vi "reward_behavior_0_6s_post_stim_timeout.vi"() -> ()   [LabVIEW 2019]
doc: "The myRIO Project template acquires acceleration data from the onboard accelerometer and displays the changes of acceleration values in a waveform chart."
uses:
  <vilib>/Analysis/Matrix/Datatypes/RealMatrix.ctl
  <vilib>/myRIO/Common/Instrument Driver Framework/myRIO v1.0/Encoder/typedefs/Encoder Signal Mode.ctl
  <vilib>/myRIO/Instrument Drivers/Onboard IO/Encoder/typedefs/Encoder Reference.ctl
  <vilib>/myRIO/Common/Instrument Driver Framework/Utilities/typedefs/myRIO Generic Hardware Reference.ctl
  <vilib>/myRIO/Common/Instrument Driver Framework/Utilities/typedefs/Hardware Version Enum.ctl
  <vilib>/myRIO/Common/Instrument Driver Framework/Utilities/typedefs/myRIO v1.0 Reference.ctl
  <vilib>/myRIO/Common/Instrument Driver Framework/Utilities/typedefs/Generic FPGA Reference.ctl
  <vilib>/myRIO/Common/Instrument Driver Framework/myRIO v1.0/Encoder/typedefs/Encoder Channels Enum.ctl
  <vilib>/myRIO/Common/Instrument Driver Framework/myRIO v1.0/Encoder/typedefs/Encoder Configuration v1.0.ctl
  <vilib>/userdefined/High Color/nirio_resource_hc.ctl
  <vilib>/myRIO/Instrument Drivers/Onboard IO/DIO/typedefs/DIO Reference.ctl
  <vilib>/myRIO/Common/Instrument Driver Framework/myRIO v1.0/DIO/typedefs/DIO Channels List.ctl
  <vilib>/myRIO/Common/Instrument Driver Framework/myRIO v1.0/DIO/typedefs/DIO Channels Enum.ctl
  <vilib>/myRIO/Common/Instrument Driver Framework/Utilities/vis/Is FPGA Ref Available.vi
  <vilib>/myRIO/Common/Instrument Driver Framework/myRIO v1.0/Encoder/vis/myRIO v1.1 Open Encoder.vi
  <vilib>/myRIO/Instrument Drivers/Onboard IO/Encoder/vis/Read.vi
  <vilib>/myRIO/Common/Instrument Driver Framework/myRIO v1.0/DIO/vis/myRIO v1.1 Open DIO.vi
  <vilib>/myRIO/Instrument Drivers/Onboard IO/DIO/vis/Write.vi
  <vilib>/myRIO/Instrument Drivers/Onboard IO/DIO/vis/Read.vi
  <vilib>/myRIO/Common/Instrument Driver Framework/Utilities/vis/Validate Channels.vi
  <vilib>/myRIO/Common/Instrument Driver Framework/myRIO v1.0/Encoder/vis/myRIO v1.0 Reserve Encoder.vi
  <vilib>/myRIO/Common/Instrument Driver Framework/myRIO v1.0/DIO/vis/myRIO v1.0 Reserve DIO.vi
  <vilib>/myRIO/Common/Instrument Driver Framework/myRIO v1.0/Encoder/vis/myRIO v1.0 Build MUX Configuration Encoder.vi
  <vilib>/myRIO/Common/Instrument Driver Framework/myRIO v1.0/Resource Manager/vis/myRIO v1.0 Reserve Channel List.vi
  <vilib>/myRIO/Common/Instrument Driver Framework/myRIO v1.0/DIO/vis/myRIO v1.0 Build MUX Configuration DIO.vi
  <vilib>/myRIO/Common/Instrument Driver Framework/myRIO v1.0/Resource Manager/vis/myRIO v1.0 Create Configuration List.vi
  <vilib>/myRIO/Common/Instrument Driver Framework/myRIO v1.0/Resource Manager/vis/myRIO v1.0 Reserve Channel.vi
  <vilib>/myRIO/Common/Instrument Driver Framework/myRIO v1.0/Resource Manager/vis/myRIO v1.0 Unreserve Channel.vi
  <vilib>/myRIO/Common/Instrument Driver Framework/myRIO v1.0/Resource Manager/vis/myRIO v1.0 Build Mutex Name.vi
  <vilib>/Utility/VariantDataType/GetNumericInfo.vi
  <vilib>/Utility/error.llb/Error Cluster From Error Code.vi
  <vilib>/myRIO/Common/Instrument Driver Framework/myRIO v1.0/myRIO v1.1 Open.vi
  <vilib>/myRIO/Common/Instrument Driver Framework/Utilities/vis/IO Manager.vi
  <vilib>/myRIO/Common/Instrument Driver Framework/Utilities/vis/Configuration Manager.vi
  <vilib>/myRIO/Common/Instrument Driver Framework/myRIO v1.0/Resource Manager/vis/myRIO v1.0 Configure IO.vi
  <vilib>/myRIO/Common/Instrument Driver Framework/myRIO v1.0/myRIO v1.0 Close.vi
  <vilib>/myRIO/Common/Instrument Driver Framework/myRIO v1.0/Encoder/vis/myRIO v1.0 Configure Encoder.vi
  <vilib>/myRIO/Common/Instrument Driver Framework/myRIO v1.0/Encoder/vis/myRIO v1.0 Read Encoder.vi
  <vilib>/myRIO/Common/Instrument Driver Framework/myRIO v1.0/DIO/vis/myRIO v1.0 Read DIO.vi
  <vilib>/myRIO/Common/Instrument Driver Framework/myRIO v1.0/DIO/vis/myRIO v1.0 Write DIO.vi
  <vilib>/myRIO/Express VI/Onboard IO/Encoder/Encoder Express VI.xnode
  <vilib>/myRIO/Instrument Drivers/Onboard IO/Encoder/vis/myRIO Encoder Open.xnode
  <vilib>/myRIO/Express VI/Onboard IO/DI/DI Express VI.xnode
  <vilib>/myRIO/Instrument Drivers/Onboard IO/DIO/vis/myRIO DIO Open.xnode
  <vilib>/myRIO/Express VI/Onboard IO/DO/DO Express VI.xnode
  <vilib>/myRIO/Instrument Drivers/Onboard IO/Encoder/Encoder.lvlib
  <vilib>/myRIO/Instrument Drivers/Onboard IO/DIO/DIO.lvlib
  <vilib>/Analysis/Matrix/NI_Matrix.lvlib
panel:
  out "Display":bool
  out "ISI Time":dbl
  out "Rewards":u16
  out "Active Trial":bool
  out "Array temp2":T1
  out "Stimuli Loaded":bool
  out "Stim_ID":dbl[](array[numeric])
  out "Reward_mat":dbl[](array[numeric])
  out "Reward":bool=TRUE
  out "Frame clock":i32
  out "Licks":u32
  out "Lick":bool
  out "Time":dbl
  out "Stop":bool
  in  "Frames to collect":u32
  out "Overflow?":bool
  out "Counter Value":i32
  out "Velocity":dbl
  out "Velocity Plot":dbl[](graph)
  out "Velocity array":dbl[](array[numeric])
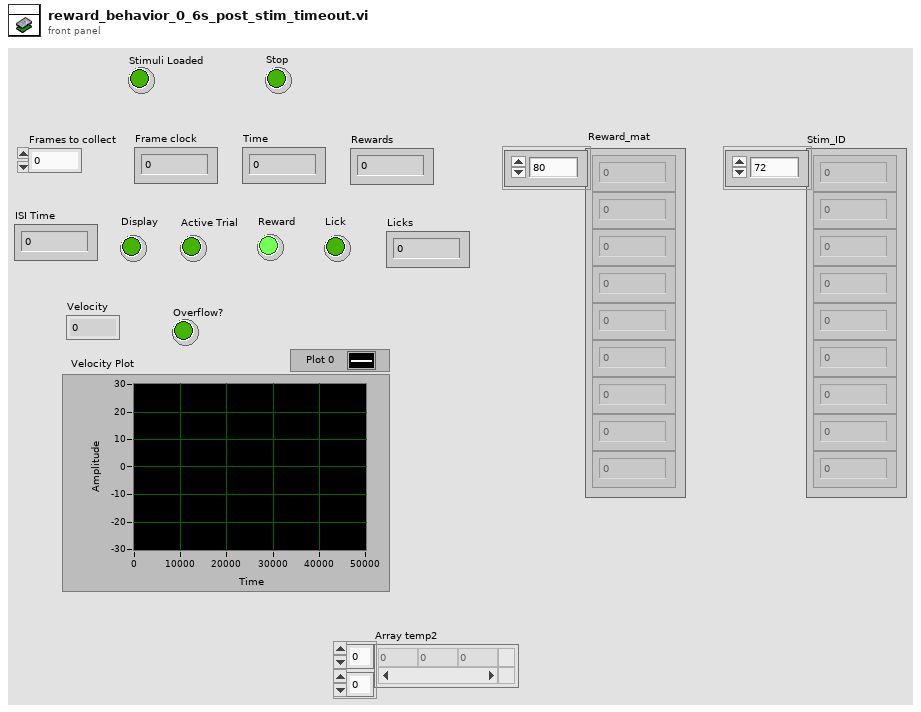
[diagram p1: front panel]
types:
  T1 = typedef "NI_Matrix.lvlib/RealMatrix.ctl" = dbl[][]
  T2 = typedef "Encoder.lvlib/Encoder Reference.ctl" = cluster{"myRIO Reference":T3, "Encoder Channels Enum":T7}
  T3 = typedef "myRIO Generic Hardware Reference.ctl" = cluster{"myRIO Model":T4, "myRIO Hardware Reference":T5}
  T4 = typedef "Hardware Version Enum.ctl" = enum16{"Unknown", "myRIO-1900", "myRIO-1950", "roboRIO", "NI ELVIS RIO CM", "ELVIS III"}
  T5 = typedef "myRIO v1.0 Reference.ctl" = cluster{"Generic FPGA Reference":T6, "Allow multiple opens":bool}
  T6 = typedef "Generic FPGA Reference.ctl" = refnum<k20>
  T7 = typedef "Encoder Channels Enum.ctl" = enum16{"Not Connected", "C/ENC0", "C/ENC1", "A/ENC", "A/ENC0", "A/ENC1", "A/ENC2", "A/ENC3", "A/ENC4", "A/ENC5", "A/ENC6", "A/ENC7", "A/ENC8", "A/ENC9", "B/ENC", "B/ENC0", "B/ENC1", "B/ENC2", "B/ENC3", "B/ENC4", "B/ENC5", "B/ENC6", "B/ENC7", "B/ENC8", "B/ENC9", "DIO/ENC0", "DIO/ENC1", "DIO/ENC2", "DIO/ENC3", "DIO/ENC4"}
  T8 = typedef "Encoder Signal Mode.ctl" = enum16{"Quadrature phase signal", "Step and direction signal"}
  T9 = typedef "nirio_resource_hc.ctl" = tag
  T10 = typedef "DIO.lvlib/DIO Reference.ctl" = cluster{"myRIO Reference":T3, "DIO Channels List":T11}
  T11 = typedef "DIO Channels List.ctl" = T12[]
  T12 = typedef "DIO Channels Enum.ctl" = enum16{"Not Connected", "C/DIO0", "C/DIO1", "C/DIO2", "C/DIO3", "C/DIO4", "C/DIO5", "C/DIO6", "C/DIO7", "A/DIO0", "A/DIO1", "A/DIO2", "A/DIO3", "A/DIO4", "A/DIO5", "A/DIO6", "A/DIO7", "A/DIO8", "A/DIO9", "A/DIO10", "A/DIO11", "A/DIO12", "A/DIO13", "A/DIO14", "A/DIO15", "A/DIO16", "A/DIO17", "A/DIO18", "A/DIO19", "B/DIO0", "B/DIO1", "B/DIO2", "B/DIO3", "B/DIO4", "B/DIO5", "B/DIO6", "B/DIO7", "B/DIO8", "B/DIO9", "B/DIO10", "B/DIO11", "B/DIO12", "B/DIO13", "B/DIO14", "B/DIO15", "B/DIO16", "B/DIO17", "B/DIO18", "B/DIO19", "LED0", "LED1", "LED2", "LED3", "Button0", "DIO/DIO0", "DIO/DIO1", "DIO/DIO2", "DIO/DIO3", "DIO/DIO4", "DIO/DIO5", "DIO/DIO6", "DIO/DIO7", "DIO/DIO8", "DIO/DIO9", "SPI/CS0", "SPI/CS1", "SPI/CS2", "SPI/CS3", "LED RADIO (Green)", "LED RADIO (Red)", "LED COMM (Green)", "LED COMM (Red)", "LED MODE (Green)", "LED MODE (Red)"}
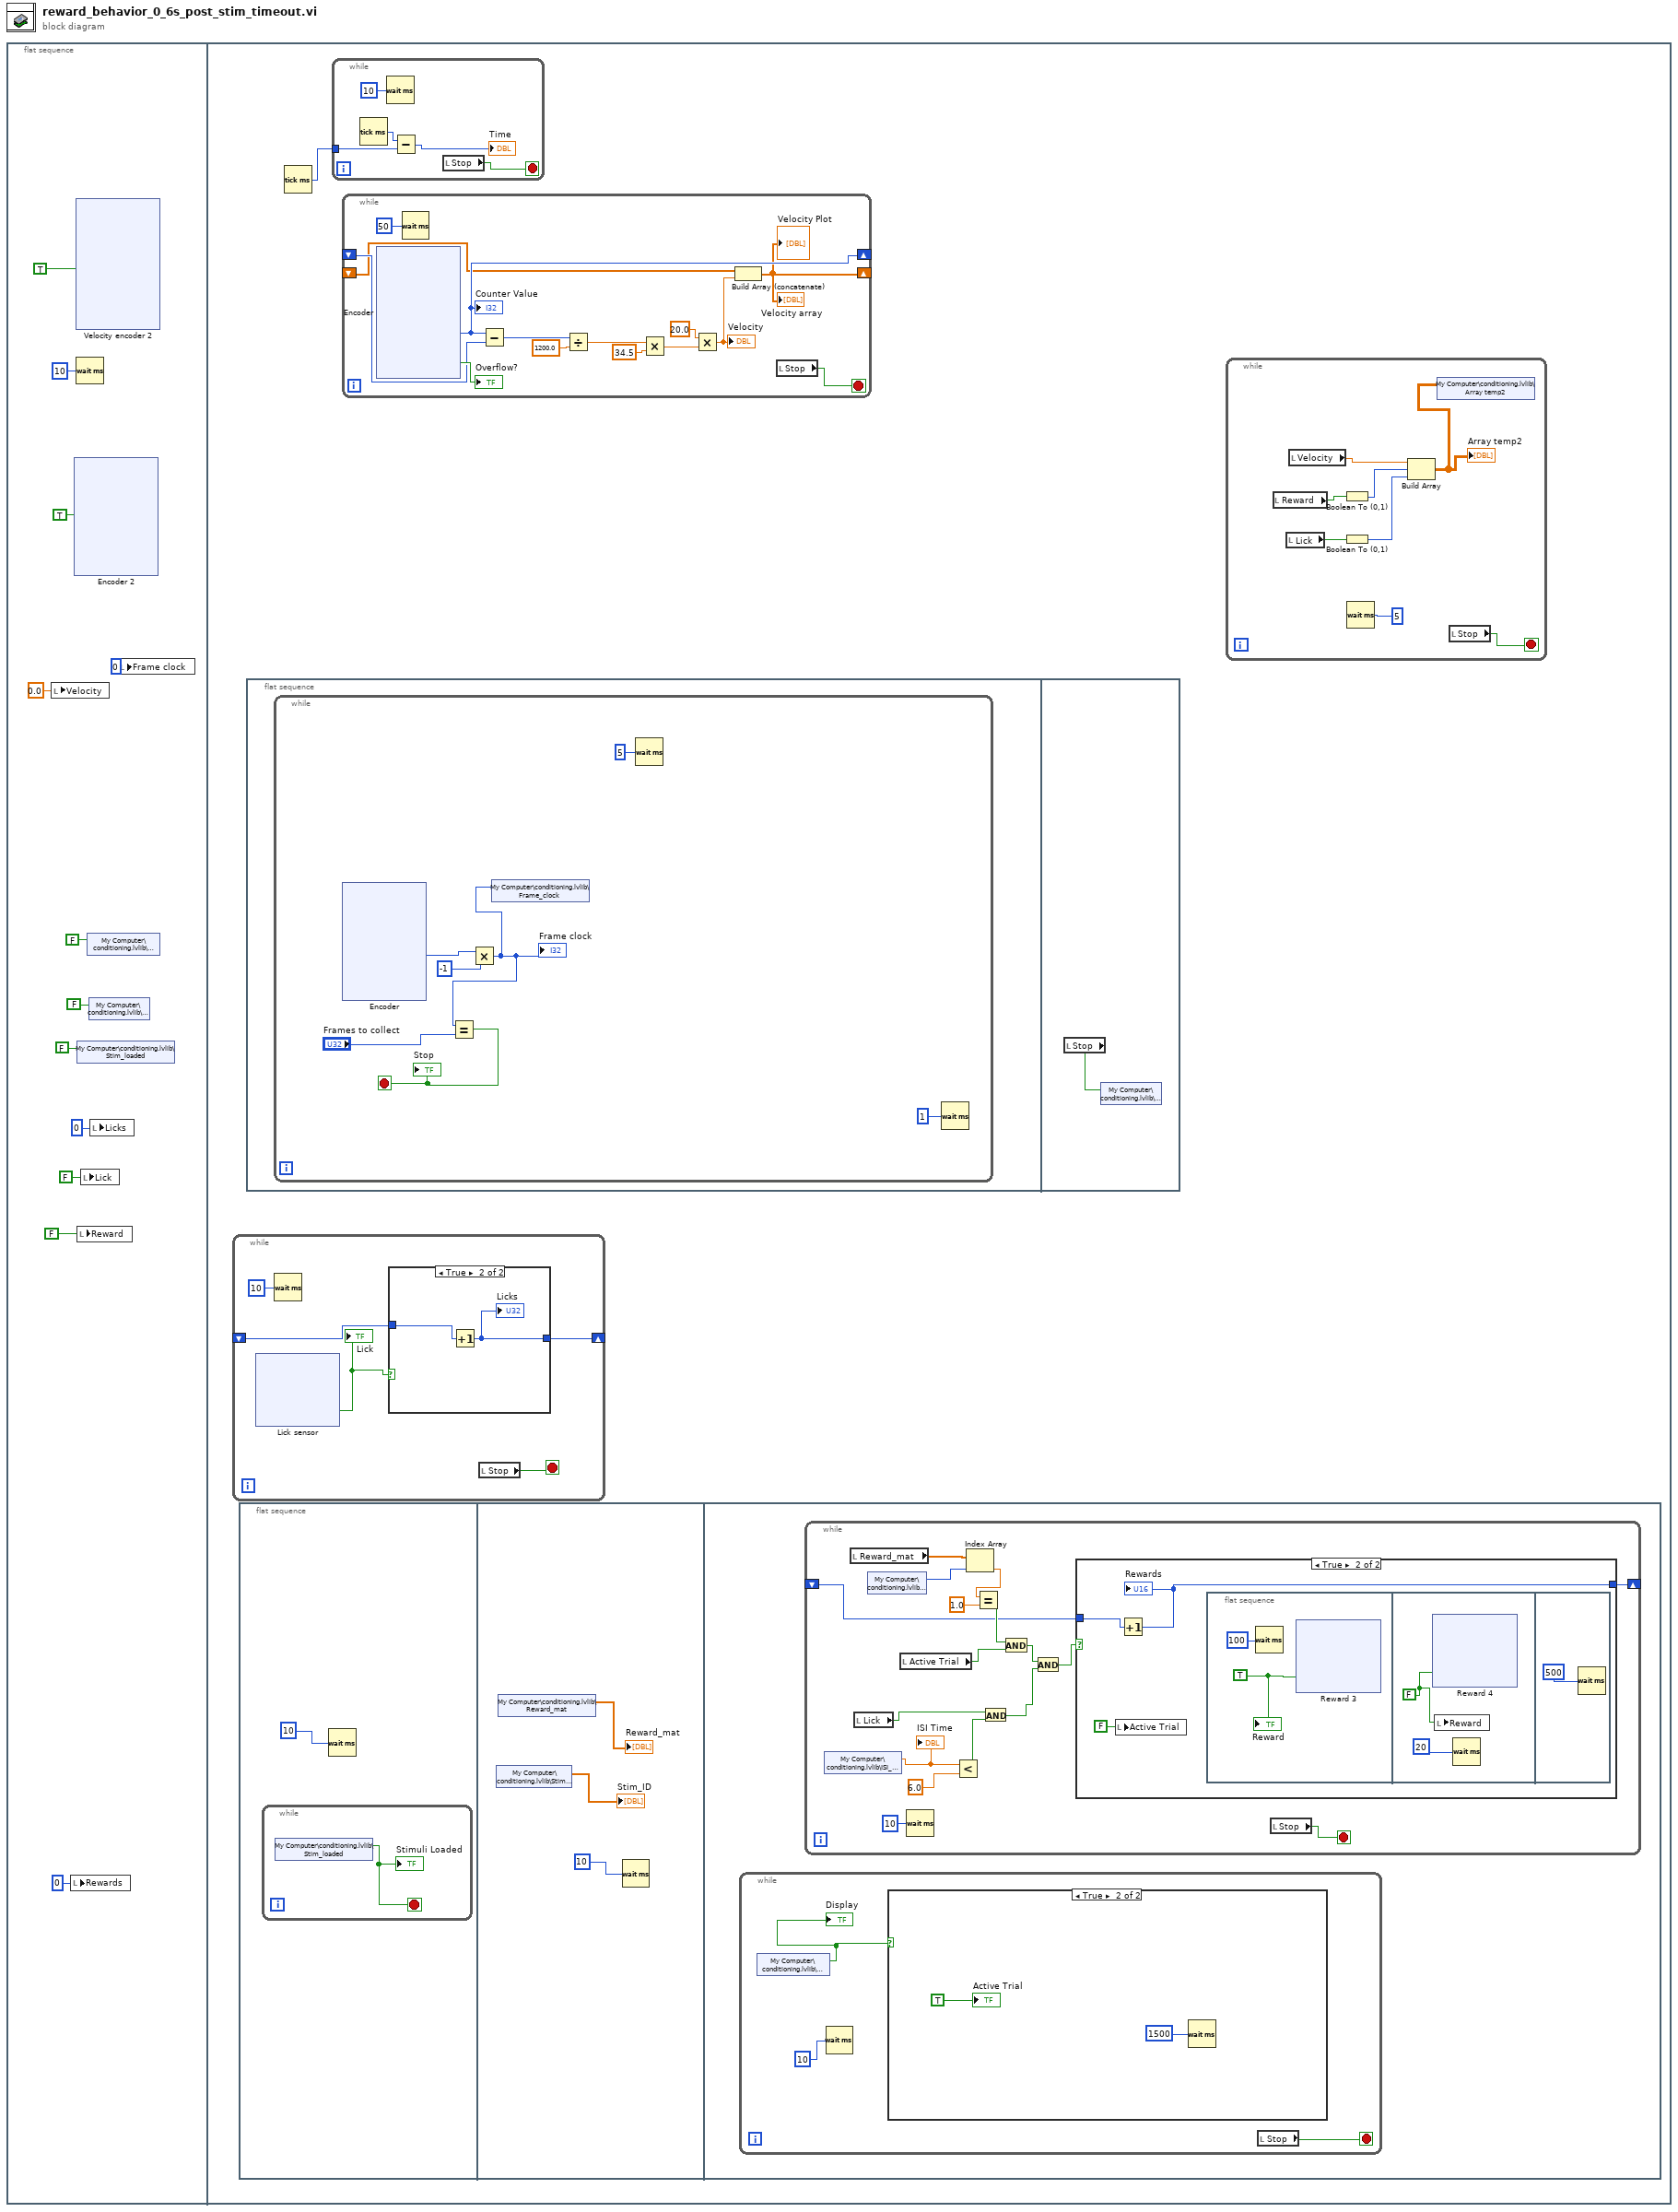
[diagram p0: block diagram]
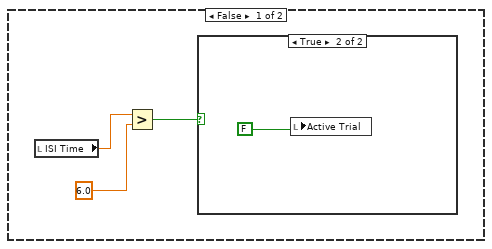
[diagram p2: hidden frame]
diagram:
  n1 = flat-sequence {
    frame #0 {
      n2 = local write "Velocity"(0.0 ("Velocity")) -> ()
      n3 = local write "Rewards"(u16 0 ("Rewards")) -> ()
      n4 = xnode "Encoder 2"("Reset Counter"=TRUE) -> ()  [unwired: 1 in, 4 out]
      n5 = xnode "Velocity encoder 2"("Reset Counter"=TRUE) -> ()  [unwired: 1 in, 4 out]
      n6 = Wait (ms)(milliseconds to wait=u32 10) -> ()  [unwired: 1 out]
      n7 = shared-variable "My Computer\\conditioning.lvlib\\Stim_loaded"(FALSE ("Stim_loaded")) -> ()  [unwired: 1 in, 1 out]
      n8 = local write "Reward"(FALSE ("Give reward")) -> ()
      n9 = local write "Lick"(FALSE ("Lick")) -> ()
      n10 = shared-variable "My Computer\\conditioning.lvlib\\Display"(FALSE ("Display")) -> ()  [unwired: 1 in, 1 out]
      n11 = shared-variable "My Computer\\conditioning.lvlib\\Stop"(FALSE ("Stop")) -> ()  [unwired: 1 in, 1 out]
      n12 = local write "Licks"(u32 0 ("Licks")) -> ()
      n13 = local write "Frame clock"(u32 0 ("Frames")) -> ()
    }
    frame #1 {
      n14 = while {
        shift-right: [w280] -> _
        shift-left: _ -> [w279]
        stop <- w278 stop-if-true
        n15 = xnode "Lick sensor"() -> ("C/DIO1 (DIO1)"=w281:bool)  [unwired: 1 in, 1 out]
        "Lick" <- w281
        n16 = Wait (ms)(milliseconds to wait=u32 10) -> ()  [unwired: 1 out]
        n17 = case shown="True" w281 {
          tunnel: [w283 w285] -> w280
          tunnel: w279 -> [w283 w284]
          frame False {
          }
          frame True {
            n18 = Increment(x=w284) -> (x+1=w285:u32)
            "Licks" <- w285
          }
        }
        n19 = local read "Stop"() -> (w278:bool)
      }
      n20 = flat-sequence {
        frame #0 {
          n21 = while {
            stop <- w115 stop-if-true
            n22 = shared-variable "My Computer\\conditioning.lvlib\\Stim_loaded"() -> (w115:bool)  [unwired: 1 in, 1 out]
            "Stimuli Loaded" <- w115
          }
          n23 = Wait (ms)(milliseconds to wait=u32 10) -> ()  [unwired: 1 out]
        }
        frame #1 {
          n24 = shared-variable "My Computer\\conditioning.lvlib\\Stim_ID"() -> (→"Stim_ID":dbl[])  [unwired: 1 in, 1 out]
          n25 = shared-variable "My Computer\\conditioning.lvlib\\Reward_mat"() -> (→"Reward_mat":dbl[])  [unwired: 1 in, 1 out]
          n26 = Wait (ms)(milliseconds to wait=u32 10) -> ()  [unwired: 1 out]
        }
        frame #2 {
          n27 = while {
            stop <- w121 stop-if-true
            n28 = shared-variable "My Computer\\conditioning.lvlib\\Display"() -> (w120:bool)  [unwired: 1 in, 1 out]
            "Display" <- w120
            n29 = Wait (ms)(milliseconds to wait=u32 10) -> ()  [unwired: 1 out]
            n30 = case shown="True" w120 {
              frame False {
                n31 = local read "ISI Time"() -> (w123:dbl)
                n32 = Greater?(x=w123, y=6.0) -> (0:w124:bool)
                n33 = case shown="True" w124 {
                  frame False {
                  }
                  frame True {
                    n34 = local write "Active Trial"(FALSE ("Active_trial")) -> ()
                  }
                }
              }
              frame True {
                n35 = Wait (ms)(milliseconds to wait=u32 1500) -> ()  [unwired: 1 out]
                "Active Trial" <- TRUE ("Active Trial")
              }
            }
            n36 = local read "Stop"() -> (w121:bool)
          }
          n37 = while {
            shift-right: [w130] -> _
            shift-left: _ -> [w129]
            stop <- w142 stop-if-true
            n38 = shared-variable "My Computer\\conditioning.lvlib\\ISI_Time"() -> (w136:dbl)  [unwired: 1 in, 1 out]
            "ISI Time" <- w136
            n39 = local read "Reward_mat"() -> (w141:dbl[])
            n40 = local read "Lick"() -> (w137:bool)
            n41 = shared-variable "My Computer\\conditioning.lvlib\\Trial"() -> (w139:u32)  [unwired: 1 in, 1 out]
            n42 = local read "Active Trial"() -> (w128:bool)
            n43 = Wait (ms)(milliseconds to wait=u32 10) -> ()  [unwired: 1 out]
            n44 = Less?(x=w136, y=6.0) -> (x < y?=w134:bool)
            n45 = Index Array(array=w141, index=w139) -> (element=w140:dbl)
            n46 = Equal?(x=w140, y=1.0) -> (x = y?=w143:bool)
            n47 = And(x=w137, y=w134) -> (x .and. y?=w133:bool)
            n48 = And(x=w143, y=w128) -> (x .and. y?=w132:bool)
            n49 = And(x=w132, y=w133) -> (x .and. y?=w131:bool)
            n50 = case shown="True" w131 {
              tunnel: [w145 w148] -> w130
              tunnel: w129 -> [w145 w147]
              frame False {
              }
              frame True {
                n51 = local write "Active Trial"(FALSE ("Active Trial")) -> ()
                n52 = Increment(x=w147) -> (x+1=w148:u16)
                "Rewards" <- w148
                n53 = flat-sequence {
                  frame #0 {
                    w149 = TRUE ("C/DIO0 (DIO0)")
                    n54 = Wait (ms)(milliseconds to wait=u32 100) -> ()  [unwired: 1 out]
                    n55 = xnode "Reward 3"("C/DIO0 (DIO0)"=w149) -> ()  [unwired: 1 in, 1 out]
                    "Reward" <- w149
                  }
                  frame #1 {
                    w187 = FALSE ("C/DIO0 (DIO0)")
                    n56 = xnode "Reward 4"("C/DIO0 (DIO0)"=w187) -> ()  [unwired: 1 in, 1 out]
                    n57 = local write "Reward"(w187) -> ()
                    n58 = Wait (ms)(milliseconds to wait=u32 20) -> ()  [unwired: 1 out]
                  }
                  frame #2 {
                    n59 = Wait (ms)(milliseconds to wait=u32 500) -> ()  [unwired: 1 out]
                  }
                }
              }
            }
            n60 = local read "Stop"() -> (w142:bool)
          }
        }
      }
      n61 = flat-sequence {
        frame #0 {
          n62 = while {
            stop <- w225 stop-if-true
            n63 = xnode "Encoder"() -> ("Counter Value"=w229:i32)  [unwired: 2 in, 3 out]
            n64 = Multiply(x=w229, y=-1) -> (x*y=w224:i32)
            "Frame clock" <- w224
            n65 = Equal?(x=w224, y="Frames to collect") -> (x = y?=w225:bool)
            "Stop" <- w225
            n66 = shared-variable "My Computer\\conditioning.lvlib\\Frame_clock"(w224) -> ()  [unwired: 1 in, 1 out]
            n67 = Wait (ms)(milliseconds to wait=u32 5) -> ()  [unwired: 1 out]
            n68 = Wait (ms)(milliseconds to wait=u32 1) -> ()  [unwired: 1 out]
          }
        }
        frame #1 {
          n69 = local read "Stop"() -> (w277:bool)
          n70 = shared-variable "My Computer\\conditioning.lvlib\\Stop"(w277) -> ()  [unwired: 1 in, 1 out]
        }
      }
      n71 = Tick Count (ms)() -> (millisecond timer value=w105:u32)
      n72 = while {
        tunnel: w105 -> [w384]
        stop <- w381 stop-if-true
        n73 = Tick Count (ms)() -> (millisecond timer value=w385:u32)
        n74 = Wait (ms)(milliseconds to wait=u32 10) -> ()  [unwired: 1 out]
        n75 = Subtract(x=w385, y=w384) -> (x-y=→"Time":u32)
        n76 = local read "Stop"() -> (w381:bool)
      }
      n77 = while {
        shift-right: [w331] -> _
        shift-left: _ -> [w332]
        shift-right: [w323] -> _
        shift-left: _ -> [w322]
        stop <- w321 stop-if-true
        n78 = xnode "Encoder"() -> ("Counter Value"=w331:i32, "Overflow?"=→"Overflow?":bool)  [unwired: 2 in, 2 out]
        "Counter Value" <- w331
        n79 = Wait (ms)(milliseconds to wait=u32 50) -> ()  [unwired: 1 out]
        n80 = Subtract(x=w331, y=w332) -> (x-y=w324:i32)
        n81 = Divide(x=w324, y=1200.0 ("600")) -> (x/y=w329:dbl)
        n82 = Multiply(x=w329, y=34.5) -> (x*y=w327:dbl)
        n83 = Multiply(x=20.0, y=w327) -> (x*y=w325:dbl)
        "Velocity" <- w325
        n84 = Build Array (concatenate)(w322, w325) -> (w323:dbl[])
        "Velocity Plot" <- w323
        "Velocity array" <- w323
        n85 = local read "Stop"() -> (w321:bool)
      }
      n86 = while {
        stop <- w107 stop-if-true
        n87 = local read "Reward"() -> (w112:bool)
        n88 = local read "Lick"() -> (w113:bool)
        n89 = local read "Velocity"() -> (w111:dbl)
        n90 = Boolean To (0,1)(Boolean=w112) -> (0, 1=w110:i16)
        n91 = Boolean To (0,1)(Boolean=w113) -> (0, 1=w109:i16)
        n92 = Wait (ms)(milliseconds to wait=u32 5) -> ()  [unwired: 1 out]
        n93 = Build Array(w111, w110, w109) -> (w106:T1)
        "Array temp2" <- w106
        n94 = shared-variable "My Computer\\conditioning.lvlib\\Array temp2"(w106) -> ()  [unwired: 1 in, 1 out]
        n95 = local read "Stop"() -> (w107:bool)
      }
    }
  }
